vi "AK Befehl mit Informationen.vi"(10 "AK Befehl":string) -> (2 "String für schreiben":string)   [LabVIEW 2020, in "FT-IR.lvlib" / "AK-Interface.lvlib"]
uses:
  AK-Interface.lvlib
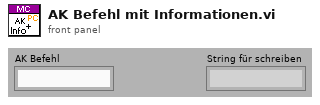
[diagram p1: front panel]
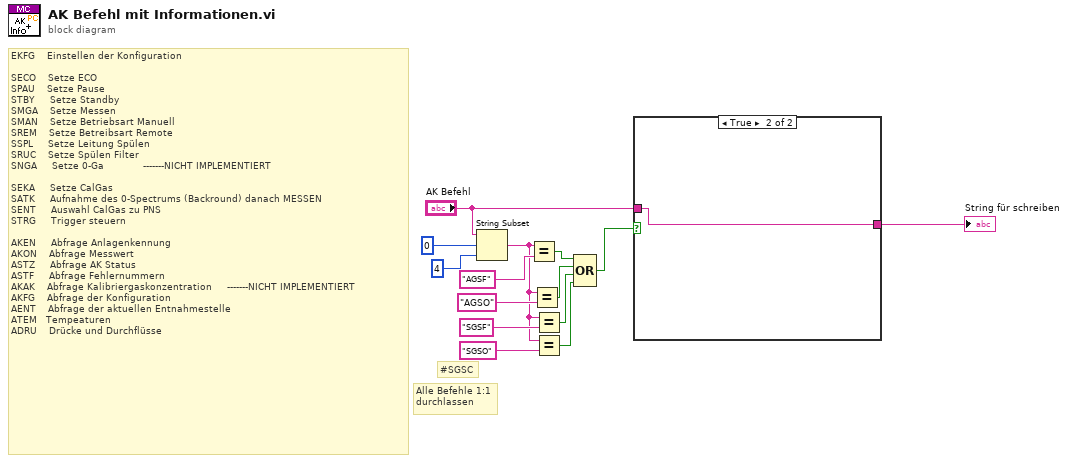
[diagram p0: block diagram]
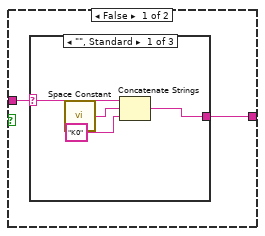
[diagram p2: hidden frame]
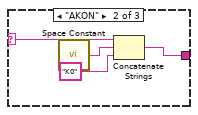
[diagram p3: hidden frame]
diagram:
  # "Alle Befehle 1:1\ndurchlassen"
  # "#SGSC"
  # "EKFG    Einstellen der Konfiguration\n\nSECO    Setze ECO\nSPAU    Setze Pause\nSTBY     Setze Standby\nSMGA    Setze Messen\nSMAN    Setze Betriebsart Manuell\nSREM    Setze Betreibsart Remote\nSSPL     Setze Leitung Spülen\nSRUC    Setze Spülen Filter\nSNGA     Setze 0-Ga             -------NICHT IMPLEMENTIERT\n\nSEKA     Setze CalGas\nSATK     Aufnahme des 0-Spectrums (Backround) danach MESSEN\nSENT     Auswahl CalGas zu PNS\nSTRG     Trigger steuern\n\nAKEN     Abfrage Anlagenkennung\nAKON    Abfrage Messwert\nASTZ     Abfrage AK Status\nASTF     Abfrage Fehlernummern\nAKAK    Abfrage Kalibriergaskonzentration     -------NICHT IMPLEMENTIERT\nAKFG    Abfrage der Konfiguration\nAENT    Abfrage der aktuellen Entnahmestelle\nATEM   Tempeaturen\nADRU    Drücke und Durchflüsse"
  n1 = String Subset(string="AK Befehl", offset (0)=0 ("Offset (0)"), length (rest)=4 ("Länge (Rest)")) -> (substring=w3:string)
  n2 = Equal?(x=w3, y="AGSF") -> (x = y?=w8:bool)
  n3 = Equal?(x=w3, y="AGSO") -> (x = y?=w7:bool)
  n4 = Equal?(x=w3, y="SGSF") -> (x = y?=w2:bool)
  n5 = Equal?(x=w3, y="SGSO") -> (x = y?=w1:bool)
  n6 = Compound Arithmetic op=OR ("Mehrfacharithmetik")(w8, w7, w2, w1) -> (w6:bool)
  n7 = case shown="True" w6 {
    tunnel: [w16 w26] -> w14
    tunnel: "AK Befehl" -> [w15 w26]
    frame False {
      n8 = case shown="\"\", Standard" w15 {
        selector: w15 -> [w18 w24 w25]
        tunnel: [w17 w21 w25] -> w16
        frame "", Default {
          n9 = call <vilib>:"Space Constant.vi"() -> ("String"=w20:string)
          n10 = Concatenate Strings(w18, w20, "K0" ("String")) -> (w17:string)
        }
        frame "AKON" {
          n11 = call <vilib>:"Space Constant.vi"() -> ("String"=w23:string)
          n12 = Concatenate Strings(w24, w23, "K0" ("String")) -> (w21:string)
        }
        frame "SFLO K0 STOP" {
        }
      }
    }
    frame True {
    }
  }
  "String für schreiben" <- w14
